vi "Zadanie2.vi"() -> ()   [LabVIEW 2012]
panel:
  out "Temperatura w st C obliczona na podstawie rezystancji:":dbl
  in  "Podaj wartoœæ rezystancji opornika platynowego:":dbl
  # "Program oblicza temperaturê na podstawie wartoœci rezystancji opornika platynoweg"
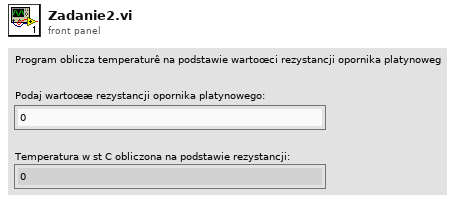
[diagram p1: front panel]
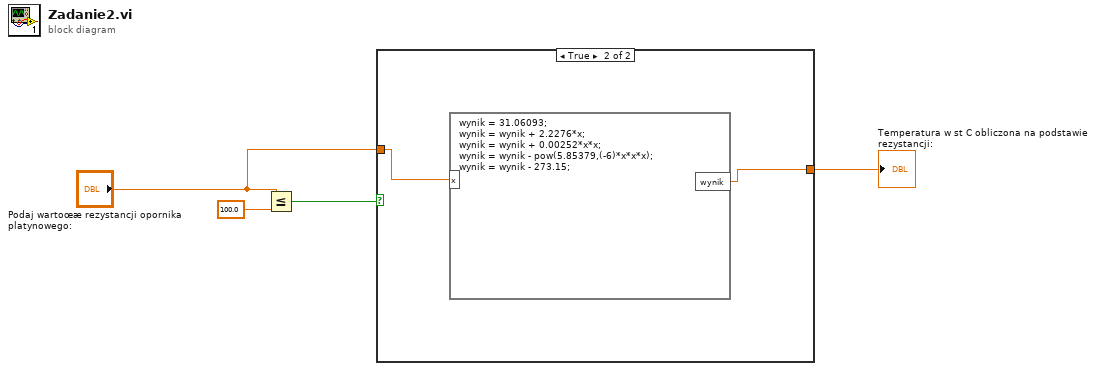
[diagram p0: block diagram]
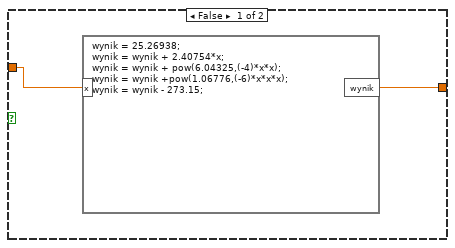
[diagram p2: hidden frame]
diagram:
  n1 = Less Or Equal?(x="Podaj wartoœæ rezystancji opornika platynowego:", y=100.0) -> (x <= y?=w3:bool)
  n2 = case shown="True" w3 {
    tunnel: "Podaj wartoœæ rezystancji opornika platynowego:" -> [w6 w7]
    tunnel: [w5 w8] -> w1
    frame False {
      n3 = formula code="wynik = 25.26938;\nwynik = wynik + 2.40754*x;\nwynik = wynik + pow(6.04325,(-4)*x*x);\nwynik = wynik +pow(1.06776,(-6)*x*x*x);\nwynik = wynik - 273.15;"("x"=w6) -> ("wynik"=w5:dbl)
    }
    frame True {
      n4 = formula code="wynik = 31.06093;\nwynik = wynik + 2.2276*x;\nwynik = wynik + 0.00252*x*x;\nwynik = wynik - pow(5.85379,(-6)*x*x*x);\nwynik = wynik - 273.15;"("x"=w7) -> ("wynik"=w8:dbl)
    }
  }
  "Temperatura w st C obliczona na podstawie rezystancji:" <- w1
